vi "Step Core.vi"(8 "error in (no error)":errorcluster, 11 "IIP3 Calculation in":refnum<class "IIP3Calculation.lvclass">) -> (0 "error out":errorcluster, 3 "IIP3 Calculation out":refnum<class "IIP3Calculation.lvclass">)   [LabVIEW 2018, in "IIP3Calculation.lvlib" / "IIP3Calculation.lvclass"]
uses:
  IIP3Calculation.lvclass
  C:/Sequence Automation/Plugins/Measurement Interface.lvlibp/Measurement Interface.lvclass
  Plugins/Measurement Interface.lvlibp/Private Methods/Measurement Name/Read Measurement Name.vi
  Plugins/Measurement Interface.lvlibp/Public Methods/Sequence Reference/Read Sequence Reference.vi
  Plugins/Measurement Interface.lvlibp/Measurement Interface.lvclass
  Plugins/TestStand API Tools (TSAT).lvlibp/Step Actions/TSAT Step Actions.lvlib
  Plugins/TestStand API Tools (TSAT).lvlibp/Sequence Actions/TSAT Sequence Actions.lvlib
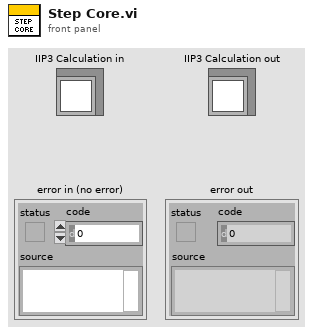
[diagram p1: front panel]
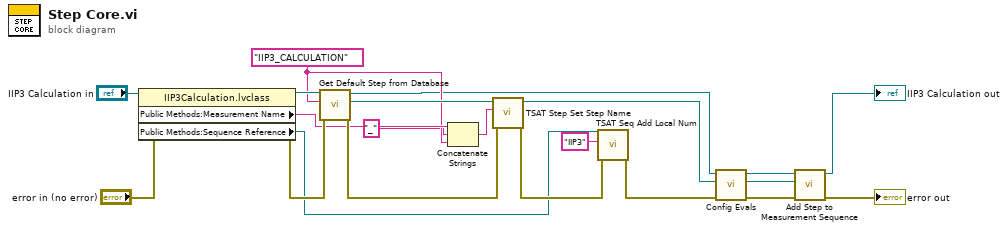
[diagram p0: block diagram]
diagram:
  w14 = "IIP3_CALCULATION" ("Default Step")
  n1 = property class="IIP3Calculation.lvclass"(reference="IIP3 Calculation in", error in="error in (no error)") -> (reference out=w16:refnum<class "IIP3Calculation.lvclass">, error out=w18:errorcluster, "Public Methods:Measurement Name"=w15:string, "Public Methods:Sequence Reference"=w9:refnum<k7>)
  n2 = call "Get Default Step from Database.vi"("error in (no error)"=w18, "Default Step"=w14, "Measurement Interface in"=w16) -> ("error out"=w19:errorcluster, "Cloned Step"=w20:refnum<k7>, "Measurement Interface out"=w6:refnum<class "IIP3Calculation.lvclass">)  [unwired: 6 in]
  n3 = Concatenate Strings(w15, "_" ("string"), w14) -> (w12:string)
  n4 = call "TSAT Step Set Step Name.vi"("Error In"=w19, "Name"=w12, "Step In"=w20) -> ("Error Out"=w11:errorcluster, "Step Out"=w1:refnum<k7>)  [unwired: 7 in]
  n5 = call "TSAT Seq Add Local Num.vi"("Error In"=w11, "Local Variable Name"="IIP3", "Sequence In"=w9) -> ("Error Out"=w10:errorcluster)  [unwired: 7 in, 1 out]
  n6 = call "Config Evals.vi"("error in (no error)"=w10, "Step In"=w1, "IIP3 Calculation in"=w6) -> ("error out"=w7:errorcluster, "Step Out"=w2:refnum<k7>, "IIP3 Calculation out"=w4:refnum<class "IIP3Calculation.lvclass">)  [unwired: 6 in]
  n7 = call "Add Step to Measurement Sequence.vi"("error in (no error)"=w7, "Step to Add"=w2, "Measurement Interface in"=w4) -> ("error out"=→"error out":errorcluster, "Measurement Interface out"=→"IIP3 Calculation out":refnum<class "IIP3Calculation.lvclass">)  [unwired: 7 in]
